vi "TemplateModule.CreateRequests.vi"(8 "error in (no error)":errorcluster) -> (0 "error out":errorcluster, 3 "Requests":T1)   [LabVIEW 2024, in "TemplateModule.lvclass"]
uses:
  TemplateModule.lvclass
  TemplateModule.lvclass/TemplateModule.ctl
  Request Events--cluster.ctl
  Do Something Args.ctl
  JQMHCore/Module/Reply.ctl
  JQMHCore/Module/RQMHModule.lvclass
  JamesT Args.ctl
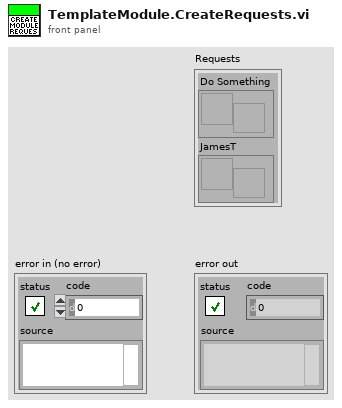
[diagram p1: front panel]
types:
  T1 = typedef "TemplateModule.lvclass/Request Events--cluster.ctl" = cluster{"Do Something":refnum<user-event>, "JamesT":refnum<user-event>}
  T2 = typedef "TemplateModule.lvclass/JamesT Args.ctl" = cluster{"Boolean":bool}
  T3 = typedef "RQMHModule.lvclass/Reply.ctl" = cluster{"Expects Reply":bool, "Reply":refnum<notifier>}
  T4 = typedef "TemplateModule.lvclass/Do Something Args.ctl" = cluster{"Msg":string}
  T5 = cluster{"Do Something Args":T4, "Reply Payload":T3}
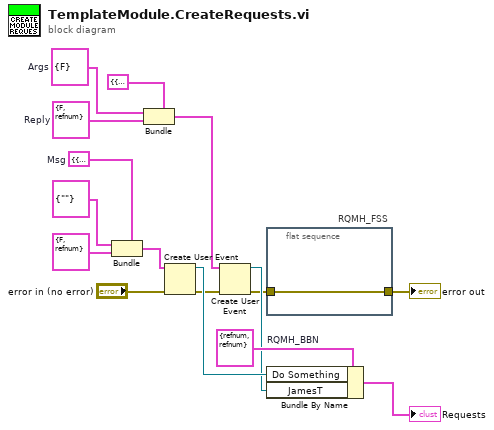
[diagram p0: block diagram]
diagram:
  w7 = T2 {"Boolean"=FALSE}  # Args
  w6 = T3 {"Expects Reply"=FALSE, "Reply"=refnum}  # Reply
  w10 = T5 {"Do Something Args"={"Msg"=""}, "Reply Payload"={"Expects Reply"=FALSE, "Reply"=refnum}}  # Msg
  n1 = Bundle(cluster=w10, "Do Something Args"=T4 {"Msg"=""}, "Reply Payload"=T3 {"Expects Reply"=FALSE, "Reply"=refnum}) -> (w13:T5)
  n2 = Bundle(cluster=cluster{"Args":T2, "Reply":T3} {"Args"={"Boolean"=FALSE}, "Reply"={"Expects Reply"=FALSE, "Reply"=refnum}} ("Msg"), "Args"=w7, "Reply"=w6) -> (w5:cluster{"Args":T2, "Reply":T3})
  n3 = Create User Event(user event datatype=w13, error in="error in (no error)") -> (user event=w9:refnum<user-event>, error out=w3:errorcluster)
  n4 = Create User Event(user event datatype=w5, error in=w3) -> (user event=w2:refnum<user-event>, error out=w1:errorcluster)
  n5 = flat-sequence "RQMH_FSS" {
    tunnel: [w17] -> w8
    tunnel: w1 -> [w17]
    frame #0 {
    }
  }
  n6 = Bundle By Name "RQMH_BBN"(cluster=T1 {"Do Something"=refnum, "JamesT"=refnum} ("Requests"), "Do Something"=w9, "JamesT"=w2) -> (→"Requests":T1)
  "error out" <- w8
